vi "findlips012.vi"(0 "Image Path":path=path "D:/图像夹/3.jpg", 7 "error in":errorcluster) -> (20 "Image":T1(plugin-control), 27 "error out":errorcluster)   [LabVIEW 2017]
doc: "Creates, and edits acquisitions using the NI Vision Acquisition Express VI.\n\nThe NI Vision Acquisition Wizard is launched by placing the Express VI on the block diagram. Select an acquisition source and configure an acquisition using NI-IMAQ, NI-IMAQdx, or simulate an acquisition by reading an AVI or image files from a folder. After an acquisition is configured, select controls and indicators to be able to programmatically set in LabVIEW. Double-click the Vision Acquisition Express VI to edit the acquisition.\n\nNote: Any images created by the Express VI need to be disposed after use. Use the IMAQ Dispose.vi to cleanup the images output by the Express VI when they are no longer needed."
uses:
  <vilib>/vision/driver/Vision Acquisition Express Utility VIs.llb/Vision Acquisition Path Convert (Path).vi
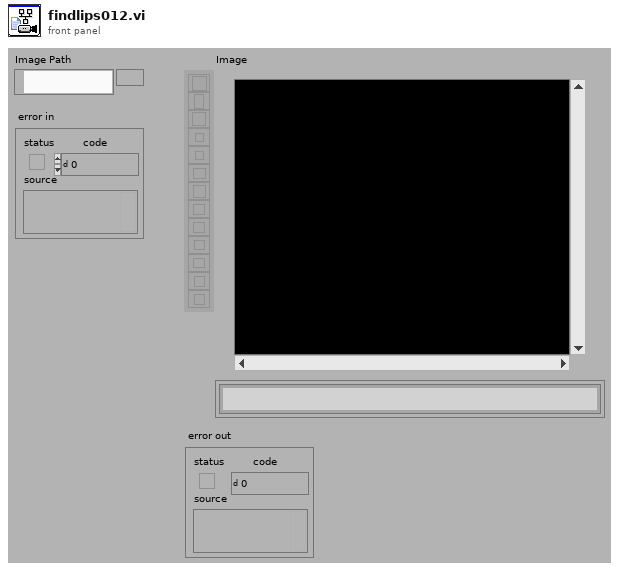
[diagram p1: front panel]
types:
  T1 = typedef "IMAQ Image.ctl" = refnum<image>
  T2 = typedef "Image Type" = u32
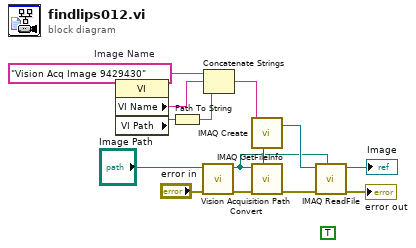
[diagram p0: block diagram]
diagram:
  (unwired) TRUE
  w5 = "Vision Acq Image 9429430"  # Image Name
  n1 = property class="VI"() -> ("VI Name"=w7:string, "VI Path"=w8:path)  [unwired: 2 in, 2 out]
  n2 = Path To String(path=w8) -> (string=w6:string)
  n3 = call-poly <vilib>:"Vision Acquisition Path Convert.vi"("Path In"="Image Path") -> ("Path Out"=w1:path)  [unwired: 10 in]
  n4 = Concatenate Strings(w5, w7, w6) -> (w4:string)
  n5 = call "IMAQ GetFileInfo"("error in (no error)"="error in", "File Path"=w1) -> ("error out"=w9:errorcluster, "Image Type"=w11:T2)  [unwired: 8 out]
  n6 = call "IMAQ Create"("Image Name"=w4, "Image Type"=w11) -> ("New Image"=w13:T1)  [unwired: 2 in, 2 out]
  n7 = call "IMAQ ReadFile"("File Path"=w1, "error in (no error)"=w9, "Image"=w13) -> ("error out"=→"error out":errorcluster, "Image Out"=→"Image":T1)  [unwired: 2 in, 5 out]
